vi "Create All Message Queues.vi"(8 "error in (no error)":errorcluster) -> (0 "error out":errorcluster, 3 "Message Queues out":T1)   [LabVIEW 2015, in "Message Queue.lvlib"]
doc: "This VI creates and initializes all the message queues for your application. If your application requires more than one message queue, right-click the \"Message Queues\" constant above and select Open Type Def. Add the new Message Queue(s) to the type definition, then initialize them in this VI."
uses:
  Message Queue.lvlib
  All Message Queues.ctl
  Message Cluster.ctl
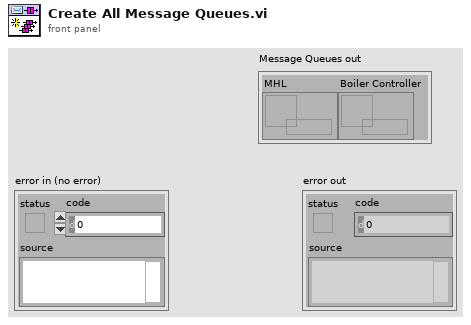
[diagram p1: front panel]
types:
  T1 = typedef "Message Queue.lvlib/All Message Queues.ctl" = cluster{"MHL":refnum<queue>, "Boiler Controller":refnum<queue>}
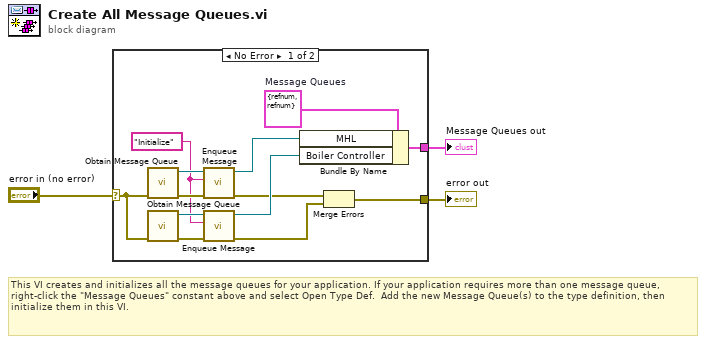
[diagram p0: block diagram]
diagram:
  # "This VI creates and initializes all the message queues for your application. If your application requires more than one message queue, right-click the \"Message Queues\" constant above and select Open Type Def.  Add the new Message Queue(s) to the type definition, then initialize them in this VI."
  n1 = case shown="No Error" "error in (no error)" {
    selector: "error in (no error)" -> [w11 w16]
    tunnel: [w7 w16] -> w3
    tunnel: [w14 _] -> w2
    frame No Error {
      w4 = "Initialize" ("Message")
      w15 = T1 {"MHL"=refnum, "Boiler Controller"=refnum}  # Message Queues
      n2 = call "Obtain Message Queue.vi"("error in (no error)"=w11) -> ("error out"=w13:errorcluster, "Message Queue"=w12:refnum<queue>)  [unwired: 9 in]
      n3 = call "Obtain Message Queue.vi"("error in (no error)"=w11) -> ("error out"=w8:errorcluster, "Message Queue"=w10:refnum<queue>)  [unwired: 9 in]
      n4 = call "Enqueue Message.vi"("error in (no error)"=w13, "Message"=w4, "Message Queue"=w12) -> ("error out"=w6:errorcluster)  [unwired: 7 in, 1 out]
      n5 = call "Enqueue Message.vi"("error in (no error)"=w8, "Message"=w4, "Message Queue"=w10) -> ("error out"=w5:errorcluster, "dup Message Queue"=w9:refnum<queue>)  [unwired: 7 in]
      n6 = Bundle By Name(cluster=w15, "MHL"=w12, "Boiler Controller"=w9) -> (w14:T1)
      n7 = Merge Errors(w6, w5) -> (w7:errorcluster)
    }
    frame Error {
    }
  }
  "Message Queues out" <- w2
  "error out" <- w3
